vi "Palettes.vi"(8 "error in (no error)":errorcluster) -> (0 "error out":errorcluster)   [LabVIEW 2021, in "Markdown.lvlib"]
doc: "Export palette images from the VI Tree SubVI positions on the block diagram. Use a square decoration to create sub-palettes."
uses:
  Markdown.lvlib
  TypeDefs/Item.ctl
  Global.vi
  <vilib>/Utility/error.llb/Error Cluster From Error Code.vi
  <vilib>/ErrorRing/Error Ring.xnode
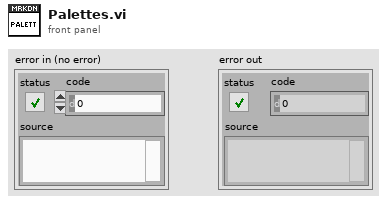
[diagram p1: front panel]
types:
  T1 = typedef "Markdown.lvlib/Item.ctl" = cluster{"Name":string, "Icon":picture, "Path":path, "Title":string, "Desc":string, "ConPane":picture, "TypeString":string, "ProjectItem":string, "VI Type":enum32{"invalid VI type", "Standard VI", "Control VI", "Global VI", "Polymorphic VI", "Configuration VI", "SubSystem", "Facade VI", "Method VI", "Statechart Diagram VI"}}
  T2 = cluster{"Left":i32, "Top":i32, "Right":i32, "Bottom":i32}
  T3 = cluster{"Name":string, "Icon":picture, "Items":T1[][]}
  T4 = typedef "LVPositionTypeDef.ctl" = cluster{"Left":i32, "Top":i32}
  T5 = typedef "LVBoundsTypeDef.ctl" = cluster{"Width":u32, "Height":u32}
  T6 = typedef "imagedata.ctl" = cluster{"image type":i32, "image depth":i32, "image":u8[], "mask":u8[], "colors":u32[], "Rectangle":cluster{"left":i16, "top":i16, "right":i16, "bottom":i16}}
  T7 = cluster{"Left":i32, "Top":i32, "Right":i32, "Bottom":i32}[]
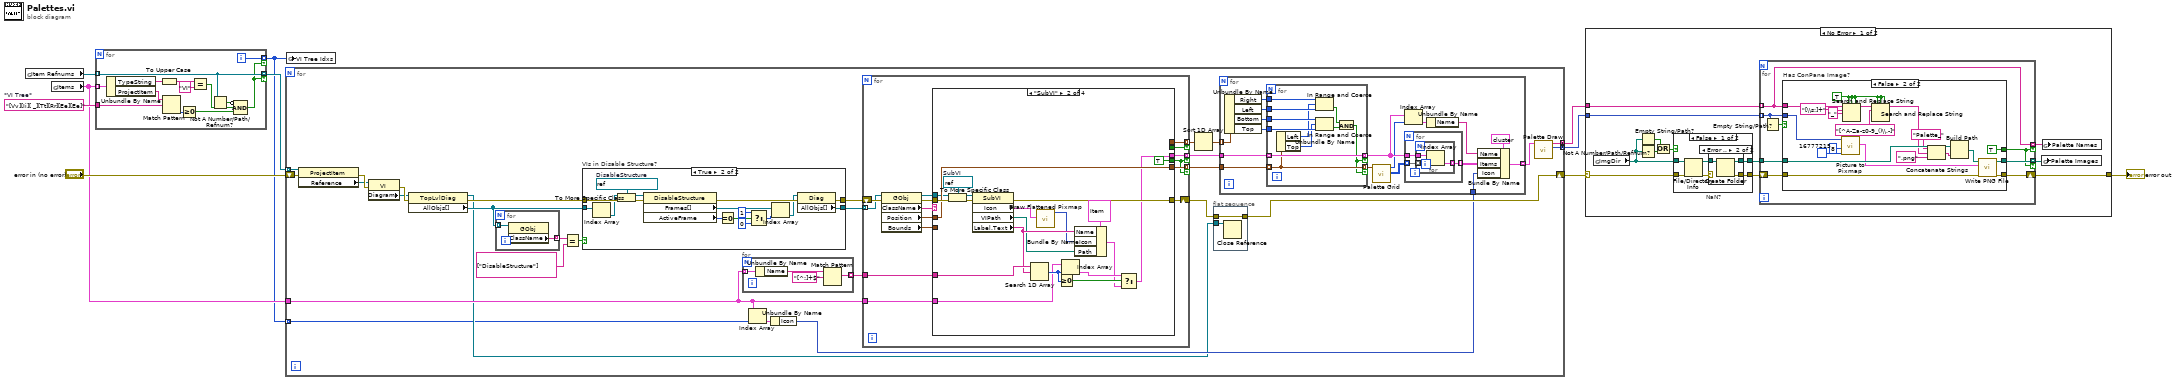
[diagram p0: block diagram]
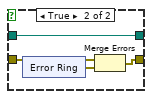
[diagram p3: hidden frame]
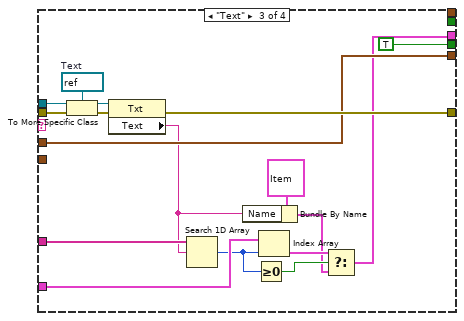
[diagram p8: hidden frame]
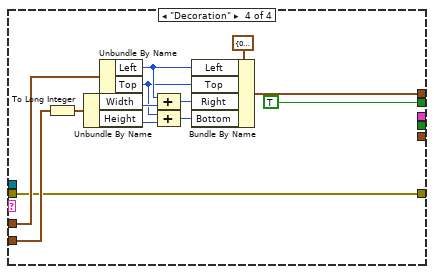
[diagram p9: hidden frame]
diagram:
  w10 = "[Vv][Ii][ _][Tt][Rr][Ee][Ee]"  # *VI Tree*
  n1 = global read "Global.vi" "Item Refnums"() -> (w3:refnum<vi>[])
  n2 = global read "Global.vi" "Items"() -> (w2:T1[])
  n3 = for {
    tunnel: w2 -> [w23] mode=indexing
    tunnel: w10 -> [w21]
    tunnel: [w13] -> w9 mode=indexing if=w11
    tunnel: w3 -> [w13] mode=indexing
    tunnel: [w12] -> w1 mode=indexing if=w11
    i -> [w12]
    n4 = Unbundle By Name(w23) -> ("TypeString"=w18:string, "ProjectItem"=w20:string)
    n5 = To Upper Case(1:w18) -> (0:w17:string)
    n6 = Match Pattern(string=w20, regular expression=w21) -> (offset past match=w22:i32)  [unwired: 1 in, 3 out]
    n7 = Greater Or Equal To 0?(x=w22) -> (x >= 0?=w19:bool)
    n8 = Equal?(x=w17, y="VI") -> (x = y?=w15:bool)
    n9 = Not A Number/Path/Refnum?(number/path/refnum=w13) -> (NaN/Path/Refnum?=w14:bool)
    n10 = Compound Arithmetic op=AND(invert w14, w15, w19) -> (w11:bool)
  }
  n11 = for {
    tunnel: w2 -> [w48]
    shift-right: [w51] -> w8
    shift-left: "error in (no error)" -> [w50]
    tunnel: [w27] -> w5 mode=concatenating
    tunnel: [w26] -> w6 mode=concatenating
    tunnel: w1 -> [w25] mode=indexing
    tunnel: w9 -> [w24] mode=indexing
    n12 = property class="ProjectItem"(reference=w24, error in=w50) -> (error out=w47:errorcluster, "Reference"=w45:refnum<vi>)  [unwired: 1 out]
    n13 = property class="VI"(reference=w45, error in=w47) -> (error out=w46:errorcluster, "Diagram"=w44:refnum<vi>)  [unwired: 1 out]
    n14 = property class="TopLvlDiag"(reference=w44, error in=w46) -> (reference out=w29:refnum<vi>, error out=w43:errorcluster, "AllObjs[]"=w38:refnum<vi>[])
    n15 = for {
      tunnel: w38 -> [w77] mode=indexing
      tunnel: [w76] -> w40 mode=indexing
      n16 = property class="GObj"(reference=w77) -> ("ClassName"=w76:string)  [unwired: 1 in, 2 out]
    }
    n17 = Equal?(x=w40, y=string[] ["DisableStructure"]) -> (x = y?=w39:bool)
    n18 = case "VIs in Disable Structure?" shown="True" w39 {
      tunnel: w43 -> [w59 w75]
      tunnel: [w59 w62] -> w42
      tunnel: [w58 w61] -> w41
      tunnel: w38 -> [w58 w60]
      frame False {
      }
      frame True {
        w72 = refnum<vi> refnum  # DisableStructure
        n19 = Index Array(array=w60) -> (element=w74:refnum<vi>)  [unwired: 1 in]
        n20 = To More Specific Class(target class=w72, reference=w74, error in=w75) -> (specific class reference=w73:refnum<vi>, error out=w71:errorcluster)
        n21 = property class="DisableStructure"(reference=w73, error in=w71) -> (error out=w70:errorcluster, "Frames[]"=w69:refnum<vi>[], "ActiveFrame"=w68:i16)  [unwired: 1 out]
        n22 = Equal To 0?(x=w68) -> (x = 0?=w67:bool)
        n23 = Select(t=1 ("index"), s=w67, f=0 ("index")) -> (s? t:f=w64:i32)
        n24 = Index Array(array=w69, index=w64) -> (element=w63:refnum<vi>)
        n25 = property class="Diag"(reference=w63, error in=w70) -> (error out=w62:errorcluster, "AllObjs[]"=w61:refnum<vi>[])  [unwired: 1 out]
      }
    }
    n26 = for {
      tunnel: w48 -> [w56] mode=indexing
      tunnel: [w55] -> w32 mode=indexing
      n27 = Unbundle By Name(w56) -> ("Name"=w54:string)
      n28 = Match Pattern(string=w54, regular expression="[^:]+$") -> (match substring=w55:string)  [unwired: 1 in, 3 out]
    }
    n29 = Index Array(array=w48, index=w25) -> (element=w31:T1)
    n30 = Unbundle By Name(w31) -> ("Icon"=w30:picture)
    n31 = for {
      tunnel: w41 -> [w91] mode=indexing
      shift-right: [w89] -> w28
      shift-left: w42 -> [w92]
      tunnel: [w82] -> w36 mode=indexing if=w83
      tunnel: [w86] -> w35 mode=indexing if=w83
      tunnel: [w85] -> w34 mode=indexing if=w84
      tunnel: w32 -> [w79]
      tunnel: w48 -> [w78]
      n32 = property class="GObj"(reference=w91, error in=w92) -> (reference out=w88:refnum<vi>, error out=w90:errorcluster, "ClassName"=w87:string, "Position"=w81:T4, "Bounds"=w80:T5)
      n33 = case shown="\"SubVI\"" w87 {
        tunnel: w90 -> [w93 w112 w129 w131]
        tunnel: [w93 w105 w128 w131] -> w89
        tunnel: w88 -> [_ w109 w125 _]
        tunnel: [_ TRUE TRUE _] -> w83
        tunnel: [_ w111 w127 _] -> w86
        tunnel: [_ _ _ w135] -> w85
        tunnel: [_ _ _ TRUE] -> w84
        tunnel: [_ w94 w117 _] -> w82
        tunnel: w81 -> [_ w111 w127 w133]
        tunnel: w80 -> [_ _ _ w132]
        tunnel: w79 -> [_ w101 w122 _]
        tunnel: w78 -> [_ w100 w121 _]
        frame Default {
        }
        frame "SubVI" {
          w108 = refnum<vi> refnum  # SubVI
          n34 = To More Specific Class(target class=w108, reference=w109, error in=w112) -> (specific class reference=w107:refnum<vi>, error out=w110:errorcluster)
          n35 = property class="SubVI"(reference=w107, error in=w110) -> (error out=w105:errorcluster, "Icon"=w106:T6, "VIPath"=w95:path, "Label.Text"=w97:string)  [unwired: 1 out]
          n36 = Search 1D Array(1D array=w101, element=w97) -> (index of element=w104:i32)  [unwired: 1 in]
          n37 = call <vilib>:"Draw Flattened Pixmap.vi"("image data"=w106) -> ("new picture"=w96:picture)  [unwired: 8 in]
          n38 = Greater Or Equal To 0?(x=w104) -> (x >= 0?=w103:bool)
          n39 = Index Array(array=w100, index=w104) -> (element=w102:T1)
          n40 = Bundle By Name(cluster=T1 {"Name"="", "Icon"=bytes[0], "Path"=path "", "Title"="", "Desc"="", "ConPane"=bytes[0], "TypeString"="", "ProjectItem"="", "VI Type"=enum."invalid VI type"} ("f"), "Name"=w97, "Icon"=w96, "Path"=w95) -> (w98:T1)
          n41 = Select(t=w102, s=w103, f=w98) -> (s? t:f=w94:T1)
        }
        frame "Text" {
          w123 = refnum<vi> refnum  # Text
          n42 = To More Specific Class(target class=w123, reference=w125, error in=w129) -> (specific class reference=w124:refnum<vi>, error out=w126:errorcluster)
          n43 = property class="Txt"(reference=w124, error in=w126) -> (error out=w128:errorcluster, "Text"=w114:string)  [unwired: 1 out]
          n44 = Search 1D Array(1D array=w122, element=w114) -> (index of element=w120:i32)  [unwired: 1 in]
          n45 = Bundle By Name(cluster=T1 {"Name"="", "Icon"=bytes[0], "Path"=path "", "Title"="", "Desc"="", "ConPane"=bytes[0], "TypeString"="", "ProjectItem"="", "VI Type"=enum."invalid VI type"} ("f"), "Name"=w114) -> (w115:T1)
          n46 = Greater Or Equal To 0?(x=w120) -> (x >= 0?=w119:bool)
          n47 = Index Array(array=w121, index=w120) -> (element=w118:T1)
          n48 = Select(t=w118, s=w119, f=w115) -> (s? t:f=w117:T1)
        }
        frame "Decoration" {
          n49 = To Long Integer(number=w132) -> (32bit integer=w136:cluster{"Width":i32, "Height":i32})
          n50 = Unbundle By Name(w136) -> ("Width"=w142:i32, "Height"=w141:i32)
          n51 = Unbundle By Name(w133) -> ("Left"=w138:i32, "Top"=w137:i32)
          n52 = Compound Arithmetic op=ADD(w138, w142) -> (w139:i32)
          n53 = Compound Arithmetic op=ADD(w137, w141) -> (w140:i32)
          n54 = Bundle By Name(cluster=T2 {"Left"=0, "Top"=0, "Right"=0, "Bottom"=0} ("Rect"), "Left"=w138, "Top"=w137, "Right"=w139, "Bottom"=w140) -> (w135:T2)
        }
      }
    }
    n55 = Sort 1D Array(array=w34) -> (sorted array=w33:T7)
    n56 = flat-sequence {
      tunnel: w29 -> [w53]
      tunnel: [w52] -> w51
      tunnel: w28 -> [w52]
      frame #0 {
        n57 = Close Reference(reference=w53) -> ()  [unwired: 1 in, 1 out]
      }
    }
    n58 = for {
      tunnel: w33 -> [w160] mode=indexing
      tunnel: w36 -> [w154]
      tunnel: w35 -> [w155]
      tunnel: [w147] -> w49 mode=indexing
      tunnel: w30 -> [w145]
      n59 = Unbundle By Name(w160) -> ("Right"=w159:i32, "Left"=w158:i32, "Bottom"=w157:i32, "Top"=w156:i32)
      n60 = for {
        tunnel: w159 -> [w177]
        tunnel: w158 -> [w176]
        tunnel: w157 -> [w175]
        tunnel: w156 -> [w174]
        tunnel: w155 -> [w168] mode=indexing
        tunnel: w154 -> [w169] mode=indexing
        tunnel: [w169] -> w151 mode=indexing if=w167
        tunnel: [w168] -> w153 mode=indexing if=w167
        n61 = Unbundle By Name(w168) -> ("Left"=w171:i32, "Top"=w170:i32)
        n62 = In Range and Coerce(upper limit=w177, x=w171, lower limit=w176) -> (In Range?=w172:bool)  [unwired: 1 out]
        n63 = In Range and Coerce(upper limit=w175, x=w170, lower limit=w174) -> (In Range?=w173:bool)  [unwired: 1 out]
        n64 = And(x=w172, y=w173) -> (x .and. y?=w167:bool)
      }
      n65 = call "Palette Grid.vi"("Positions"=w153) -> ("Indexes"=w152:i32[][], "Label Index"=w150:i32)  [unwired: 9 in]
      n66 = Index Array(array=w151, index=w150) -> (element=w148:T1)
      n67 = for {
        tunnel: w152 -> [w162] mode=indexing
        tunnel: w151 -> [w163]
        tunnel: [w161] -> w149 mode=indexing
        n68 = for {
          tunnel: w163 -> [w166]
          tunnel: w162 -> [w165] mode=indexing
          tunnel: [w164] -> w161 mode=indexing
          n69 = Index Array(array=w166, index=w165) -> (element=w164:T1)
        }
      }
      n70 = Unbundle By Name(w148) -> ("Name"=w146:string)
      n71 = Bundle By Name(cluster=T3 {"Name"="", "Icon"=bytes[0], "Items"=[]} ("Palette"), "Name"=w146, "Items"=w149, "Icon"=w145) -> (w147:T3)
    }
    n72 = call "Palette Draw.vi"("Palettes"=w49) -> ("Palette Image"=w26:picture[], "Palette Names"=w27:string[])  [unwired: 9 in]
  }
  n73 = global write "Global.vi" "VI Tree Idxs"(w1) -> ()
  n74 = case shown="No Error" w8 {
    selector: w8 -> [w189 w238]
    tunnel: [w188 w238] -> w4
    tunnel: w6 -> [w182 _]
    tunnel: w5 -> [w181 _]
    frame No Error {
      n75 = global read "Global.vi" "ImgDir"() -> (w180:path)
      n76 = Empty String/Path?(string/path=w180) -> (empty?=w184:bool)
      n77 = Not A Number/Path/Refnum?(number/path/refnum=w180) -> (NaN/Path/Refnum?=w185:bool)
      n78 = Or(x=w184, y=w185) -> (x .or. y?=w183:bool)
      n79 = case "NaN?" shown="False" w183 {
        tunnel: w189 -> [w195 w204]
        tunnel: w180 -> [w193 w203]
        tunnel: [w192 w202] -> w187
        tunnel: [w190 w203] -> w186
        frame False {
          n80 = File/Directory Info(path=w193, error in=w195) -> (path out=w191:path, error out=w194:errorcluster)  [unwired: 5 out]
          n81 = case shown="Error .." w194 {
            selector: w194 -> [w196 _]
            tunnel: [w196 w200] -> w192
            tunnel: w191 -> [w197 w199]
            tunnel: [w197 w198] -> w190
            frame No Error {
            }
            frame Error {
              n82 = Create Folder(path (use dialog)=w199) -> (created path=w198:path, error out=w200:errorcluster)  [unwired: 2 in, 1 out]
            }
          }
        }
        frame True {
          n83 = xnode "Error Ring"() -> ("error out"=w201:errorcluster)
          n84 = Merge Errors(w204, w201) -> (w202:errorcluster)
        }
      }
      n85 = for {
        shift-right: [w216] -> w188
        shift-left: w187 -> [w212]
        tunnel: [w215] -> w179 mode=indexing if=w211
        tunnel: w186 -> [w214]
        tunnel: [w209] -> w178 mode=indexing if=w211
        tunnel: w182 -> [w210] mode=indexing
        tunnel: w181 -> [w209] mode=indexing
        n86 = Empty String/Path?(string/path=w210) -> (empty?=w213:bool)
        n87 = case "Has ConPane Image?" shown="False" w213 {
          tunnel: w212 -> [w217 w233]
          tunnel: [w217 w237] -> w216
          tunnel: [_ w235] -> w215
          tunnel: w214 -> [_ w234]
          tunnel: w209 -> [_ w220]
          tunnel: w210 -> [_ w222]
          tunnel: [_ TRUE] -> w211
          frame True {
          }
          frame False {
            w223 = TRUE ("replace all? (F)")
            n88 = call <vilib>:"Picture to Pixmap.vi"("Background Color"=u32 16777215, "depth"=8, "picture"=w222) -> ("image data"=w221:T6)  [unwired: 7 in, 1 out]
            n89 = Search and Replace String(replace all?=w223, case sensitive?=w223, multiline?=w223, input string=w220, search string="[\\s:]+", replace string="_" ("replace string (\"\")")) -> (result string=w226:string)  [unwired: 2 in, 3 out]
            n90 = Search and Replace String(replace all?=w223, case sensitive?=w223, multiline?=w223, input string=w226, search string="[^A-Za-z0-9_()\\.-]") -> (result string=w227:string)  [unwired: 3 in, 3 out]
            n91 = Concatenate Strings("Palette_", w227, ".png" ("string")) -> (w219:string)
            n92 = Build Path(base path=w234, name or relative path=w219) -> (appended path=w236:path)
            n93 = call <vilib>:"Write PNG File.vi"("error in (no error)"=w233, "image data"=w221, "path to PNG file"=w236) -> ("error out"=w237:errorcluster, "path"=w235:path)  [unwired: 7 in]
          }
        }
      }
      n94 = global write "Global.vi" "Palette Images"(w179) -> ()
      n95 = global write "Global.vi" "Palette Names"(w178) -> ()
    }
    frame Error {
    }
  }
  "error out" <- w4
